vi "Split strings.vi"(8 "Item Indent":i32, 10 "regular expression":string=":", 11 "qualified name":string) -> (3 "Arr":T1(array[cluster]))   [LabVIEW 2021, in "Tree.lvlib" / "Tree.lvclass"]
uses:
  Tree.lvclass
panel:
  # "Строит дерево с одним конечным элементом"
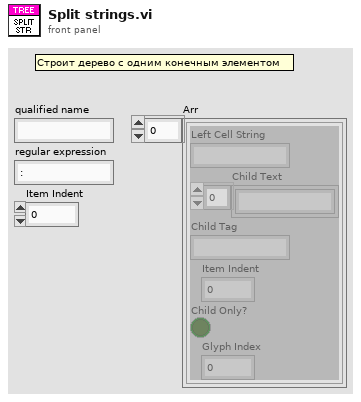
[diagram p1: front panel]
types:
  T1 = cluster{"Left Cell String":string, "Child Text":string[], "Child Tag":string, "Item Indent":i32, "Child Only?":bool, "Glyph Index":i32}[]
  T2 = cluster{"Left Cell String":string, "Child Text":string[], "Child Tag":string, "Item Indent":i32, "Child Only?":bool, "Glyph Index":i32}
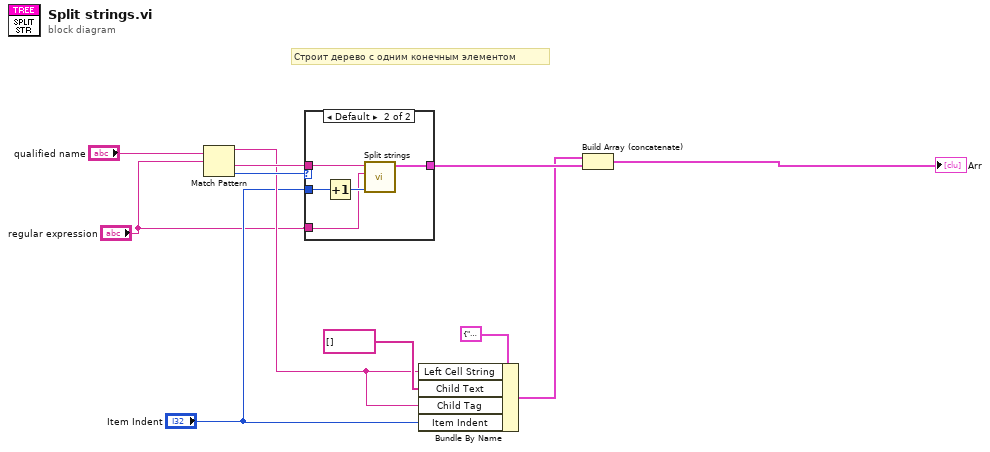
[diagram p0: block diagram]
diagram:
  # "Строит дерево с одним конечным элементом"
  n1 = Match Pattern(string="qualified name", regular expression="regular expression") -> (before substring=w5:string, after substring=w11:string, offset past match=w6:i32)  [unwired: 1 in, 1 out]
  n2 = case shown="Default" w6 {
    tunnel: w11 -> [_ w16]
    tunnel: [_ w15] -> w8
    tunnel: "Item Indent" -> [_ w14]
    tunnel: "regular expression" -> [_ w12]
    frame -1 {
    }
    frame Default {
      n3 = Increment(x=w14) -> (x+1=w13:i32)
      n4 = call "Split strings.vi"("Item Indent"=w13, "regular expression"=w12, "qualified name"=w16) -> ("Arr"=w15:T1)  [unwired: 8 in]
    }
  }
  n5 = Bundle By Name(cluster=T2 {"Left Cell String"="", "Child Text"=[], "Child Tag"="", "Item Indent"=0, "Child Only?"=FALSE, "Glyph Index"=0} ("Item"), "Left Cell String"=w5, "Child Text"=string[] [], "Child Tag"=w5, "Item Indent"="Item Indent") -> (w3:T2)
  n6 = Build Array (concatenate)(w3, w8) -> (→"Arr":T1)
